vi "AnalyzeStaticLinkages.vi"(0 "LabVIEW File to Analyze":path, 5 "Public Server Directory":path, 11 "error in":errorcluster) -> (4 "Filepath Map":cluster{"Key":string, "Filepath":path}[](array[cluster]), 15 "error out":errorcluster)   [LabVIEW 2013]
uses:
  Featherweight/Core/Error/FTW-ERR-ThrowError.vi
panel:
  # "Inputs"
  # "Debug"
  # "Outputs"
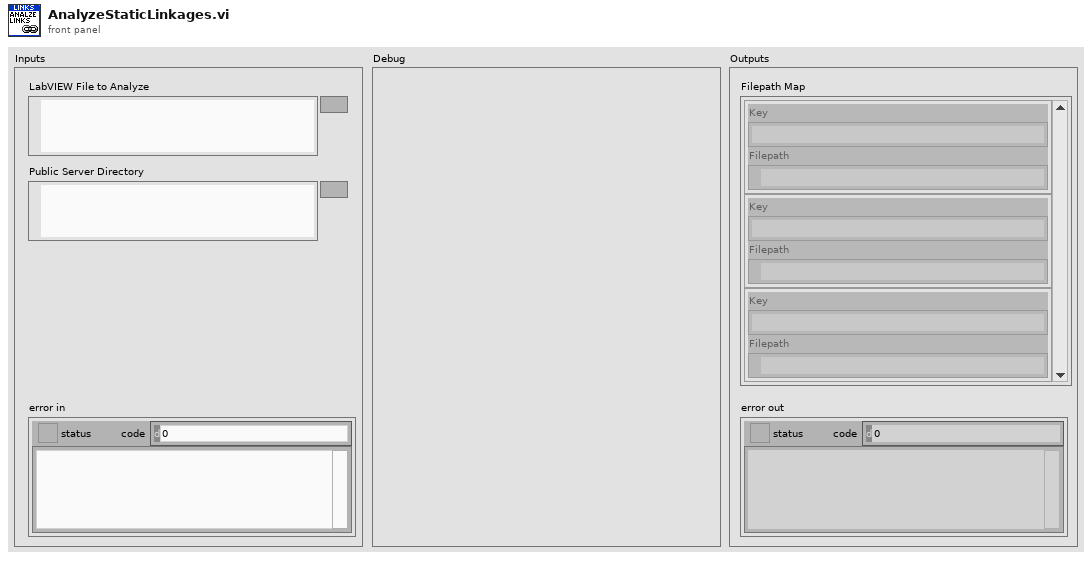
[diagram p1: front panel]
types:
  T1 = cluster{"nodes":cluster{"index":i32, "name":string, "owner":string, "collapsible":bool, "canOpen":bool, "isReentrant":bool, "isInlined":bool}[], "links":cluster{"source":i32, "target":u32, "value":i32}[]}
  T2 = typedef "FTW-Linker-LinkerInfoStructure.ctl" = cluster{"path":path, "delimited name":string, "Filetype":T3, "iState":u32, "iStyle":u16, "wStyle":u16, "buttons":u16, "viflags":u32, "viflags2":u32, "links":u32[]}
  T3 = typedef "FTW-Linker-LabVIEWFiletype.ctl" = enum32{"Invalid file", "Unknown type", "Instrument", "Control", "Polymorphic VI", "Project", "Library", "LVClass", "XControl", "XNode", "Shared library", ".NET assembly", "ActiveX interface", "CIN", "Run-time menu", "Palette menu", "Help file", "LLB", "XNode Edit Dependency", "Class Private Data Control", "Statechart", "MathScript .m file", "Ladder Diagram", "LVLibp", "XNode Build Dependency"}
  T4 = cluster{"index":i32, "name":string, "owner":string, "collapsible":bool, "canOpen":bool, "isReentrant":bool, "isInlined":bool}
  T5 = typedef "imagedata.ctl" = cluster{"image type":i32, "image depth":i32, "image":u8[], "mask":u8[], "colors":u32[], "Rectangle":cluster{"left":i16, "top":i16, "right":i16, "bottom":i16}}
  T6 = cluster{"source":i32, "target":u32, "value":i32}[]
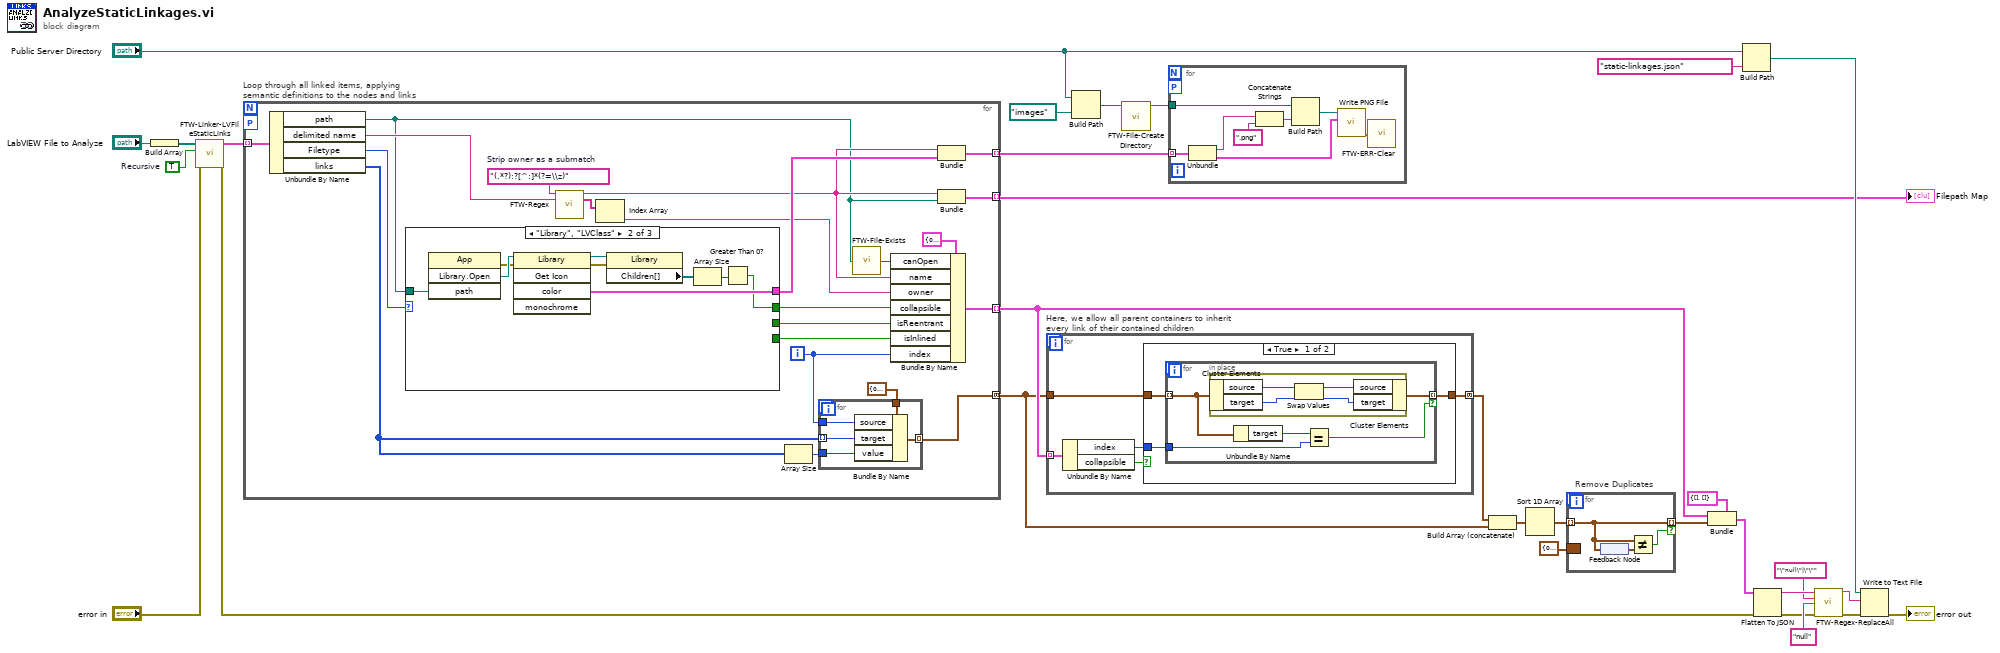
[diagram p0: block diagram]
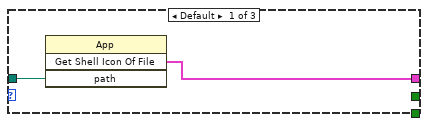
[diagram p3: hidden frame]
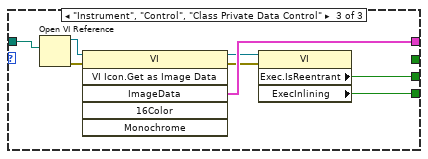
[diagram p4: hidden frame]
diagram:
  w20 = TRUE  # Recursive
  n1 = Build Array("LabVIEW File to Analyze") -> (w21:path[])
  n2 = call "FTW-Linker-LVFileStaticLinks.vi"("error in"="error in", "Recursive"=w20, "LabVIEW Files"=w21) -> ("error out"=w18:errorcluster, "LinkerInfo"=w17:T2[])  [unwired: 7 in]
  n3 = for "Loop through all linked items, applying semantic definitions to the nodes and links" {
    tunnel: w17 -> [w52] mode=indexing
    tunnel: [w51] -> w15 mode=indexing
    tunnel: [w33] -> w8 mode=concatenating
    workers-P: _ -> [_]
    tunnel: [w43] -> w3 mode=indexing
    tunnel: [w35] -> w2 mode=indexing
    i -> [w47]
    w41 = "(.*?):?[^:]*(?=\\z)"  # Strip owner as a submatch
    n4 = Unbundle By Name(w52) -> ("path"=w31:path, "delimited name"=w39:string, "Filetype"=w45:T3, "links"=w42:u32[])
    n5 = case shown="\"Library\", \"LVClass\"" w45 {
      tunnel: w31 -> [w59 w68 w76]
      tunnel: [_ w60 _] -> w38
      tunnel: [_ _ w75] -> w49
      tunnel: [_ _ w74] -> w48
      tunnel: [w58 w67 w73] -> w44
      frame Default {
        n6 = invoke class="App" method="Get Shell Icon Of File"("path"=w59) -> ("GetShellIconOfFile"=w58:T5)  [unwired: 3 in, 3 out]
      }
      frame "Library", "LVClass" {
        n7 = invoke class="App" method="Library.Open"("path"=w68) -> (error out=w65:errorcluster, "Open Library"=w66:refnum<vi>)  [unwired: 3 in, 2 out]
        n8 = invoke class="Library" method="Get Icon"(reference=w66, error in=w65) -> (reference out=w64:refnum<vi>, error out=w63:errorcluster, "color"=w67:T5)  [unwired: 3 in, 2 out]
        n9 = property class="Library"(reference=w64, error in=w63) -> ("Children[]"=w62:refnum<vi>[])  [unwired: 2 out]
        n10 = Array Size(array=w62) -> (size(s)=w61:i32)
        n11 = Greater Than 0?(x=w61) -> (x > 0?=w60:bool)
      }
      frame "Instrument", "Control", "Class Private Data Control" {
        n12 = Open VI Reference(vi path=w76) -> (vi reference=w71:refnum<vi>, error out=w72:errorcluster)  [unwired: 5 in]
        n13 = invoke class="VI" method="VI Icon.Get as Image Data"(reference=w71, error in=w72) -> (reference out=w70:refnum<vi>, error out=w69:errorcluster, "ImageData"=w73:T5)  [unwired: 4 in, 3 out]
        n14 = property class="VI"(reference=w70, error in=w69) -> ("Exec.IsReentrant"=w75:bool, "ExecInlining"=w74:bool)  [unwired: 2 out]
      }
    }
    n15 = call "FTW-Regex.vi"("Regular Expression"=w41, "Input String"=w39) -> ("Match"=w36:string, "Submatches"=w40:string[])  [unwired: 9 in, 3 out]
    n16 = Index Array(array=w40) -> (element=w32:string)  [unwired: 1 in]
    n17 = Array Size(array=w42) -> (size(s)=w46:i32)
    n18 = for {
      tunnel: w42 -> [w56] mode=indexing
      tunnel: w47 -> [w57]
      tunnel: [w54] -> w33 mode=indexing
      tunnel: w46 -> [w55]
      tunnel: cluster{"source":i32, "target":u32, "value":i32} {"source"=0, "target"=0, "value"=0} -> [w53]
      n19 = Bundle By Name(cluster=w53, "source"=w57, "target"=w56, "value"=w55) -> (w54:cluster{"source":i32, "target":u32, "value":i32})
    }
    n20 = call "FTW-File-Exists.vi"("Filepath"=w31) -> ("Exists?"=w34:bool)
    n21 = Bundle By Name(cluster=T4 {"index"=0, "name"="", "owner"="", "collapsible"=FALSE, "canOpen"=FALSE, "isReentrant"=FALSE, "isInlined"=FALSE}, "canOpen"=w34, "name"=w36, "owner"=w32, "collapsible"=w38, "isReentrant"=w49, "isInlined"=w48, "index"=w47) -> (w51:T4)
    n22 = Bundle("Match"=w36, "ImageData"=w44) -> (w35:cluster{"Match":string, "ImageData":T5})  [unwired: 1 in]
    n23 = Bundle("Match"=w36, "path"=w31) -> (w43:cluster{"Match":string, "path":path})  [unwired: 1 in]
  }
  "Filepath Map" <- w3
  n24 = for "Here, we allow all parent containers to inherit every link of their contained children" {
    tunnel: w15 -> [w80] mode=indexing
    tunnel: [w79] -> w16 mode=concatenating
    tunnel: w8 -> [w78]
    n25 = Unbundle By Name(w80) -> ("index"=w77:i32, "collapsible"=w81:bool)
    n26 = case shown="True" w81 {
      tunnel: [w82 _] -> w79
      tunnel: w78 -> [w84 _]
      tunnel: w77 -> [w83 _]
      frame True {
        n27 = for {
          tunnel: w84 -> [w86] mode=indexing
          tunnel: w83 -> [w89]
          tunnel: [w85] -> w82 mode=indexing if=w88
          n28 = in-place {
            n29 = in-place-cluster #1(w86) -> ("source"=w93:i32, "target"=w91:u32)
            n30 = Swap Values(12:w93, 14:w91) -> (1:w92:i32, 3:w90:u32)  [unwired: 1 in]
            n31 = in-place-cluster #1("source"=w92, "target"=w90) -> (w85:cluster{"source":i32, "target":u32, "value":i32})
          }
          n32 = Unbundle By Name(w86) -> ("target"=w87:u32)
          n33 = Equal?(x=w87, y=w89) -> (x = y?=w88:bool)
        }
      }
      frame False {
      }
    }
  }
  n34 = Build Path(base path="Public Server Directory", name or relative path=path "images") -> (appended path=w27:path)
  n35 = call "FTW-File-CreateDirectory.vi"("Directory to Create"=w27) -> ("Created Directory"=w19:path)  [unwired: 13 in, 1 out]
  n36 = for {
    tunnel: w19 -> [w101]
    workers-P: _ -> [_]
    tunnel: w2 -> [w94] mode=indexing
    n37 = Unbundle(w94) -> ("Match"=w96:string, "ImageData"=w99:T5)
    n38 = Concatenate Strings(w96, ".png" ("string")) -> (w97:string)
    n39 = Build Path(base path=w101, name or relative path=w97) -> (appended path=w98:path)
    n40 = call <vilib>:"Write PNG File.vi"("image data"=w99, "path to PNG file"=w98) -> ("error out"=w95:errorcluster)  [unwired: 8 in, 1 out]
    n41 = call "FTW-ERR-Clear.vi"("error to snuff"=w95) -> ()  [unwired: 1 out]
  }
  n42 = Build Array (concatenate)(w16, w8) -> (w6:T6)
  n43 = Sort 1D Array(array=w6) -> (sorted array=w7:T6)
  n44 = for "Remove Duplicates" {
    tunnel: w7 -> [w102] mode=indexing
    tunnel: [w102] -> w4 mode=indexing if=w104
    border: cluster{"source":i32, "target":u32, "value":i32} {"source"=0, "target"=0, "value"=0} -> [_]
    n45 = feedback-in #2(w102) -> ()
    n46 = feedback #2() -> (w103:cluster{"source":i32, "target":u32, "value":i32})
    n47 = Not Equal?(x=w102, y=w103) -> (x != y?=w104:bool)
  }
  n48 = Bundle(cluster=T1 {"nodes"=[], "links"=[]}, "nodes"=w15, "links"=w4) -> (w25:T1)
  n49 = Build Path(base path="Public Server Directory", name or relative path="static-linkages.json" ("Object Key")) -> (appended path=w29:path)
  n50 = Flatten To JSON(anything=w25, error in (no error)=w18) -> (JSON string=w14:string, 11:w10:errorcluster)  [unwired: 1 in]
  n51 = call "FTW-Regex-ReplaceAll.vi"("String"=w14, "Search for (Regular Expression)"="\"null\"|\"\"", "Replace with"="null" ("Search for (Regular Expression)"), "error in"=w10) -> ("String out"=w13:string, "error out"=w9:errorcluster)  [unwired: 9 in, 1 out]
  n52 = Write to Text File(file (use dialog)=w29, text=w13, error in=w9) -> (error out=→"error out":errorcluster)  [unwired: 1 in, 2 out]
